vi "SignalGenerator_x410_fxp16.vi"(10 "phase":fxp<+,64,64>, 11 "Reset":bool) -> (0 "data_valid":bool, 1 "Cos":fxp<+/-,16,0>, 2 "Sin":fxp<+/-,16,0>)   [LabVIEW 2025]
uses:
  <vilib>/rvi/IPIntegrationNode/IPINode_Typedef/niFpgaIPINodeSupportedFamilies.ctl
  <vilib>/rvi/IPIntegrationNode/IPINode_Utilities/niFpgaIPINodeSimCore.vi
  <vilib>/rvi/FXPMathLib/FxpInterpret/XNode/nifxpmath_Interpret.xnode
  <vilib>/rvi/XilinxIP/XIPIN_XNode/niFpgaXIPIN.xnode
  Xilinx/DDS_simulator/xsim.dir/DDS_Compiler_8AEA4D6678494B609559049F07B86E68/xsimk_8AEA4D6678494B609559049F07B86E68.dll
  <vilib>/rvi/IPIntegrationNode/IPINode_Xnode/niFpgaIPINode.xnode
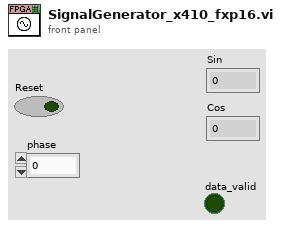
[diagram p1: front panel]
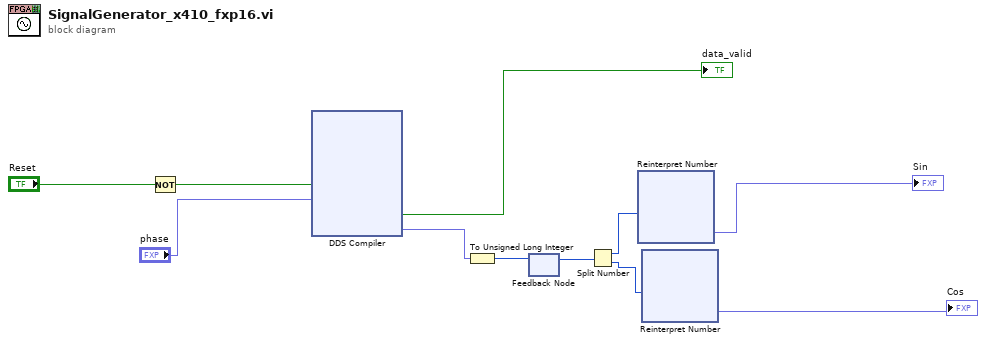
[diagram p0: block diagram]
diagram:
  n1 = Not(x="Reset") -> (.not. x?=w6:bool)
  n2 = xnode ("DDS Compiler")("aresetn"=w6, "s_axis_phase_tdata"="phase") -> ("m_axis_data_tvalid"=→"data_valid":bool, "m_axis_data_tdata"=w4:fxp<+,32,32>)  [unwired: 2 in]
  n3 = To Unsigned Long Integer(number=w4) -> (unsigned 32bit integer=w8:u32)
  n4 = feedback #1() -> (w7:u32)  [unwired: 1 in]
  n5 = feedback-in #1(w8) -> ()
  n6 = Split Number(x=w7) -> (hi(x)=w11:u16, lo(x)=w10:u16)
  n7 = xnode "Reinterpret Number"("x"=w11) -> ("y"=→"Sin":fxp<+/-,16,0>)
  n8 = xnode "Reinterpret Number"("x"=w10) -> ("y"=→"Cos":fxp<+/-,16,0>)
